vi "Read Background Data.vi"(8 "error in":errorcluster, 11 "Inset in":refnum<class "Inset.lvclass">) -> (0 "error out":errorcluster, 2 "Data":T1, 3 "Inset out":refnum<class "Inset.lvclass">)   [LabVIEW 2019, in "Inset.lvclass"]
uses:
  Inset.lvclass
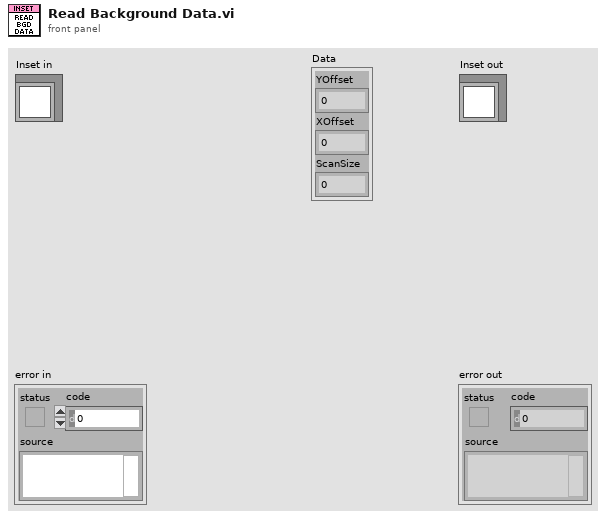
[diagram p1: front panel]
types:
  T1 = cluster{"YOffset":dbl, "XOffset":dbl, "ScanSize":dbl}
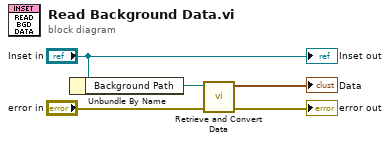
[diagram p0: block diagram]
diagram:
  n1 = Unbundle By Name("Inset in") -> ("Background Path"=w4:path)
  n2 = call "Retrieve and Convert Data.vi"("error in (no error)"="error in", "Path"=w4) -> ("error out"=→"error out":errorcluster, "Data"=→"Data":T1)  [unwired: 8 in]
  "Inset out" <- "Inset in"
